vi "WriteStartEndTimeRequest.vi"(6 "SettlingTime":dbl, 8 "error in (no error)":errorcluster, 9 "EndTime":dbl, 10 "StartTime":dbl, 11 "ModuleID":i32=-1) -> (0 "error out":errorcluster)   [LabVIEW 2014, in "WfrmPlugins.lvlib" / "BaseWfrmPlugin.lvclass"]
uses:
  BaseWfrmPlugin.lvclass
  WfrmModule/Protected/clEventType.ctl
  <vilib>/Utility/error.llb/Error Cluster From Error Code.vi
  <vilib>/ErrorRing/Error Ring.xnode
  WfrmModule/WfrmModule.lvlib
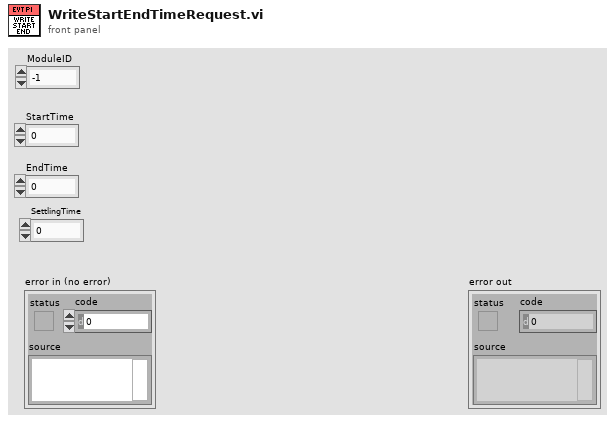
[diagram p1: front panel]
types:
  T1 = typedef "WfrmModule.lvlib/clRequestEvents.ctl" = cluster{"StopRequest":refnum<user-event>, "LoadPluginRequest":refnum<user-event>, "WriteEvtConfig":refnum<user-event>, "ReadEvtConfig":refnum<user-event>, "WriteTimeArray":refnum<user-event>, "ReadTimeArray":refnum<user-event>, "WriteEvtParams":refnum<user-event>, "ReadEvtParams":refnum<user-event>, "GetEvtReportArray":refnum<user-event>, "ReadPathToPlugin":refnum<user-event>, "GetEvtSignal":refnum<user-event>, "SendArbWfrm":refnum<user-event>, "ShowPanel":refnum<user-event>, "ReadWfrmParams":refnum<user-event>, "WriteWfrmParams":refnum<user-event>, "WriteStartEndTime":refnum<user-event>, "ConfigDlg":refnum<user-event>, "ReadStartEndSettlingTime":refnum<user-event>}
  T2 = typedef "WfrmModule.lvlib/clEventType.ctl" = cluster{"ModuleID":i32, "Data":variant}
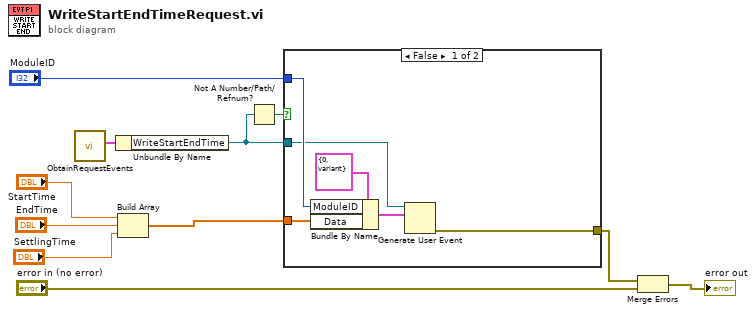
[diagram p0: block diagram]
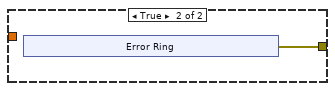
[diagram p2: hidden frame]
diagram:
  n1 = call "ObtainRequestEvents.vi"() -> ("clRequestEvents"=w7:T1)  [unwired: 10 in, 1 out]
  n2 = Unbundle By Name(w7) -> ("WriteStartEndTime"=w2:refnum<user-event>)
  n3 = Build Array("StartTime", "EndTime", "SettlingTime") -> (w4:dbl[])
  n4 = Not A Number/Path/Refnum?(number/path/refnum=w2) -> (NaN/Path/Refnum?=w3:bool)
  n5 = case shown="False" w3 {
    tunnel: w2 -> [w14 _]
    tunnel: "ModuleID" -> [w16 _]
    tunnel: w4 -> [w15 _]
    tunnel: [w12 w18] -> w8
    frame False {
      n6 = Bundle By Name(cluster=T2 {"ModuleID"=0, "Data"=variant} ("clEventType"), "ModuleID"=w16, "Data"=w15) -> (w13:T2)
      n7 = Generate User Event(user event=w14, event data cluster=w13) -> (error out=w12:errorcluster)  [unwired: 2 in, 1 out]
    }
    frame True {
      n8 = xnode "Error Ring"() -> ("error out"=w18:errorcluster)
    }
  }
  n9 = Merge Errors(w8, "error in (no error)") -> (→"error out":errorcluster)
